vi "DestroyParser.vi"(8 "error in (no error)":errorcluster, 11 "ArgumentParser in":refnum<class "ArgumentParser.lvclass">) -> (0 "error out":errorcluster)   [LabVIEW 2022 SP3, in "ArgumentParser.lvlib" / "ArgumentParser.lvclass"]
uses:
  ArgumentParser.lvclass
  ArgumentParser.lvclass/ArgumentParser.ctl
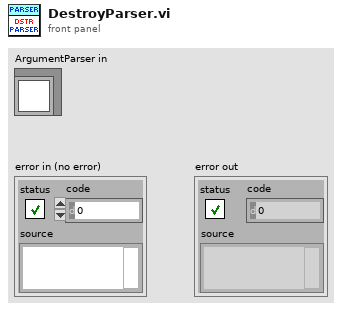
[diagram p1: front panel]
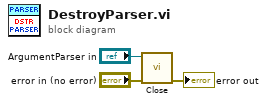
[diagram p0: block diagram]
diagram:
  n1 = call-dynamic "Close.vi"("error in (no error)"="error in (no error)", "PythonWrapper in"="ArgumentParser in") -> ("error out"=→"error out":errorcluster)  [unwired: 9 in]
